vi "Reset.vi"(8 "error in (no error)":errorcluster, 11 "DC Brick in":refnum<class "DC Brick.lvclass">) -> (0 "error out":errorcluster, 3 "DC Brick out":refnum<class "DC Brick.lvclass">)   [LabVIEW 2011, in "Tinkerforge.lvlib" / "DC Brick.lvclass"]
doc: "This VI will reset the Brick. Calling this function on a Brick inside of a stack will reset the whole stack.\n\nAfter a reset you have to create new device objects, calling functions on the existing ones will result in undefined behavior!"
uses:
  DC Brick.lvclass
  Device/Device.lvclass
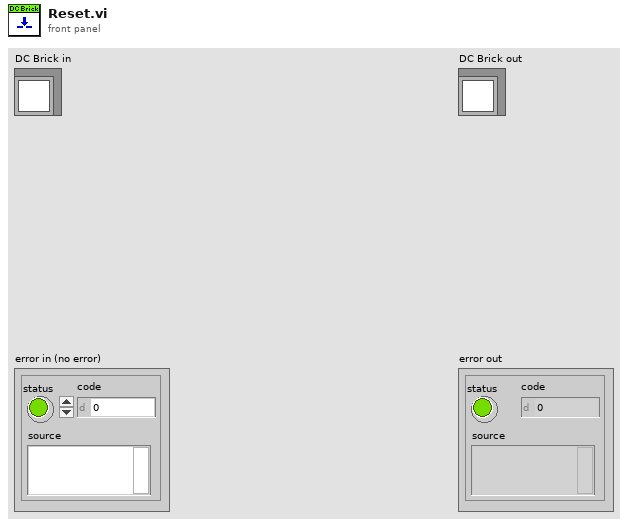
[diagram p1: front panel]
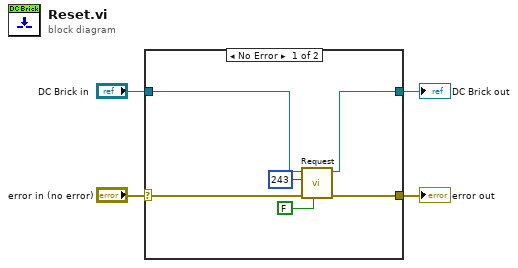
[diagram p0: block diagram]
diagram:
  n1 = case shown="No Error" "error in (no error)" {
    selector: "error in (no error)" -> [w5 w12]
    tunnel: [w6 w12] -> w3
    tunnel: [w9 w11] -> w1
    tunnel: "DC Brick in" -> [w10 w11]
    frame No Error {
      n2 = call "Request.vi"("Response"=FALSE, "error in (no error)"=w5, "Function ID"=u8 243, "Device in"=w10) -> ("error out"=w6:errorcluster, "Device out"=w9:refnum<class "DC Brick.lvclass">)  [unwired: 3 in, 3 out]
    }
    frame Error {
    }
  }
  "error out" <- w3
  "DC Brick out" <- w1
